vi "Timed Loop Running Time.vi"(10 "Counter":i32, 11 "Period (microsec)":i64) -> (3 "Time (sec)":dbl)   [LabVIEW 2018]
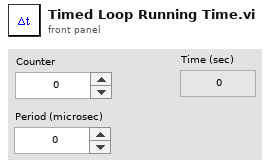
[diagram p1: front panel]
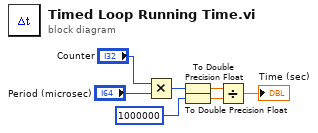
[diagram p0: block diagram]
diagram:
  n1 = Multiply(x="Counter", y="Period (microsec)") -> (x*y=w7:i64)
  n2 = To Double Precision Float(number=w7) -> (double precision float=w6:dbl)
  n3 = To Double Precision Float(number=1000000) -> (double precision float=w4:dbl)
  n4 = Divide(x=w6, y=w4) -> (x/y=→"Time (sec)":dbl)
